vi "Variant to DBL Array.vi"(8 "error in (no error)":errorcluster, 11 "Data (Variant)":variant) -> (0 "error out":errorcluster, 2 "2D Array":dbl[][](array[numeric]), 3 "1D Array":dbl[](array[numeric]))   [LabVIEW 2019, in "LV-Data.lvclass"]
uses:
  LV-Data.lvclass
  <vilib>/Utility/error.llb/Error Cluster From Error Code.vi
  <vilib>/ErrorRing/Error Ring.xnode
  <vilib>/Utility/Data Type/NI_Data Type.lvlib
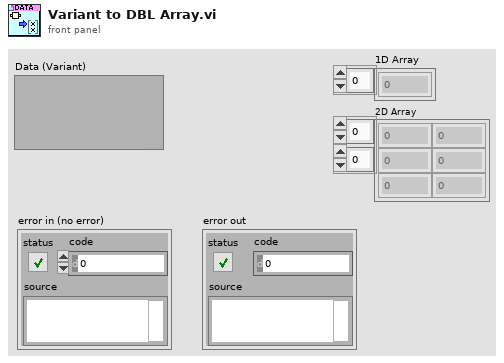
[diagram p1: front panel]
types:
  T1 = typedef "NI_Data Type.lvlib/Data Type.ctl" = enum8{"Invalid Type", "Void", "I8", "I16", "I32", "I64", "U8", "U16", "U32", "U64", "Single Float", "Double Float", "Extended Float", "Single Complex", "Double Complex", "Extended Complex", "Enum U8", "Enum U16", "Enum U32", "Enum U64", "Single Float With Unit", "Double Float With Unit", "Extended Float With Unit", "Single Complex with Unit", "Double Complex with Unit", "Extended Complex with Unit", "Boolean", "String", "Path", "Picture", "Tag", "Array", "Cluster", "Variant", "LV Variant", "Waveform", "Timestamp", "Digital Waveform", "Digital Data", "ExpressData", "Refnum", "External Data", "VI", "Poly VI", "LabVIEW Class Instance", "Fixed Point", "Set Collection", "Map Collection"}
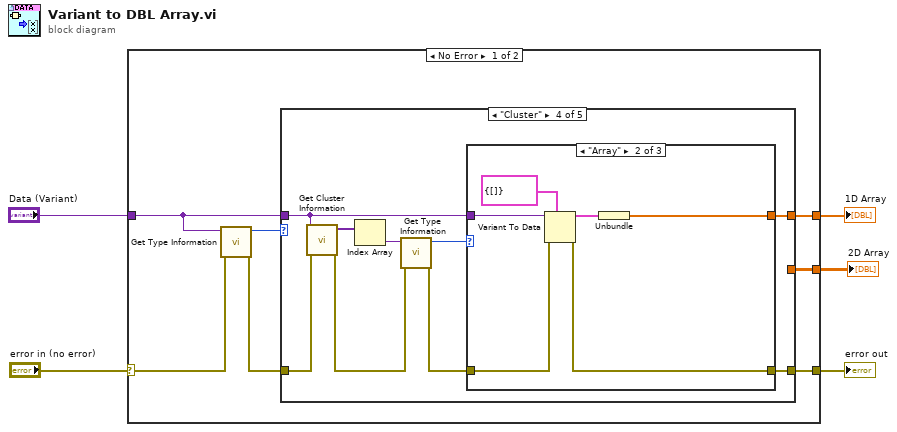
[diagram p0: block diagram]
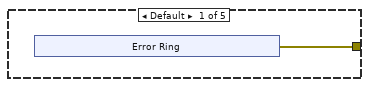
[diagram p2: hidden frame]
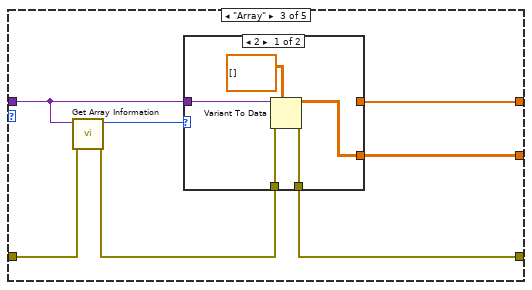
[diagram p4: hidden frame]
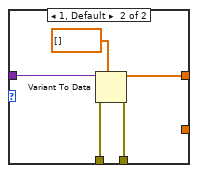
[diagram p5: hidden frame]
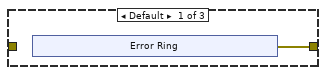
[diagram p6: hidden frame]
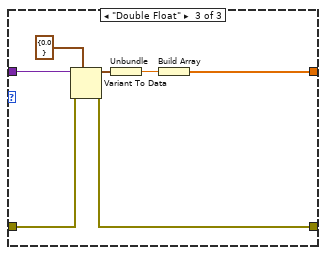
[diagram p7: hidden frame]
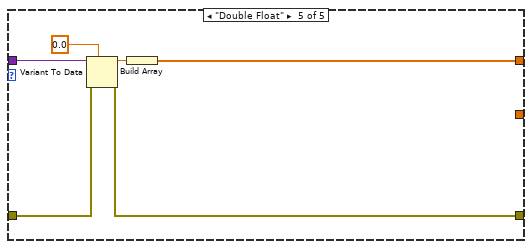
[diagram p8: hidden frame]
diagram:
  n1 = case shown="No Error" "error in (no error)" {
    selector: "error in (no error)" -> [w7 w69]
    tunnel: [w11 _] -> w5
    tunnel: [w8 w69] -> w4
    tunnel: "Data (Variant)" -> [w10 _]
    tunnel: [w6 _] -> w1
    frame No Error {
      n2 = call <vilib>:"Get Type Information.vi"("error in (no error)"=w7, "variant"=w10) -> ("error out"=w9:errorcluster, "type"=w12:T1)  [unwired: 5 in, 3 out]
      n3 = case shown="\"Cluster\"" w12 {
        tunnel: [w13 w18 w25 w39 w63] -> w8
        tunnel: [_ _ w20 w36 w65] -> w11
        tunnel: w10 -> [_ _ w24 w37 w67]
        tunnel: w9 -> [_ w18 w23 w44 w64]
        tunnel: [_ _ w19 _ _] -> w6
        frame Default {
          n4 = xnode "Error Ring"() -> ("error out"=w13:errorcluster)
        }
        frame "Void" {
        }
        frame "Array" {
          n5 = call <vilib>:"Get Array Information.vi"("error in (no error)"=w23, "variant"=w24) -> ("error out"=w22:errorcluster, "number of dimensions"=w21:i32)  [unwired: 6 in, 2 out]
          n6 = case shown="2" w21 {
            tunnel: [w29 w34] -> w25
            tunnel: w24 -> [w28 w33]
            tunnel: w22 -> [w27 w32]
            tunnel: [_ w31] -> w20
            tunnel: [w26 _] -> w19
            frame 2 {
              n7 = Variant To Data(error in=w27, type=dbl[][] [], Variant=w28) -> (data=w26:dbl[][], error out=w29:errorcluster)
            }
            frame 1, Default {
              n8 = Variant To Data(error in=w32, type=dbl[] [], Variant=w33) -> (data=w31:dbl[], error out=w34:errorcluster)
            }
          }
        }
        frame "Cluster" {
          n9 = call <vilib>:"Get Cluster Information.vi"("error in (no error)"=w44, "variant"=w37) -> ("error out"=w41:errorcluster, "cluster elements"=w43:variant[])  [unwired: 8 in]
          n10 = Index Array(array=w43) -> (element=w42:variant)  [unwired: 1 in]
          n11 = call <vilib>:"Get Type Information.vi"("error in (no error)"=w41, "variant"=w42) -> ("error out"=w40:errorcluster, "type"=w38:T1)  [unwired: 5 in, 3 out]
          n12 = case shown="\"Array\"" w38 {
            tunnel: [w45 w53 w59] -> w39
            tunnel: [_ w51 w61] -> w36
            tunnel: w40 -> [_ w54 w60]
            tunnel: w37 -> [_ w50 w56]
            frame Default {
              n13 = xnode "Error Ring"() -> ("error out"=w45:errorcluster)
            }
            frame "Array" {
              n14 = Variant To Data(error in=w54, type=cluster{dbl[]} {[]}, Variant=w50) -> (data=w55:cluster{dbl[]}, error out=w53:errorcluster)
              n15 = Unbundle(w55) -> (w51:dbl[])
            }
            frame "Double Float" {
              n16 = Variant To Data(error in=w60, type=cluster{dbl} {0.0}, Variant=w56) -> (data=w62:cluster{dbl}, error out=w59:errorcluster)
              n17 = Unbundle(w62) -> (w57:dbl)
              n18 = Build Array(w57) -> (w61:dbl[])
            }
          }
        }
        frame "Double Float" {
          n19 = Variant To Data(error in=w64, type=0.0, Variant=w67) -> (data=w68:dbl, error out=w63:errorcluster)
          n20 = Build Array(w68) -> (w65:dbl[])
        }
      }
    }
    frame Error {
    }
  }
  "1D Array" <- w5
  "error out" <- w4
  "2D Array" <- w1
